vi "TypeConv.vi"(6 "Manifestation Ancestor Path":path, 7 "Action":T2, 8 "Type Path":path, 9 "Alternative Name":string, 10 "Category":T1, 11 "Type Name":string) -> (0 "Has Projection?":bool, 1 "Projection Out":string, 2 "Param Writer":refnum<class "Abstract Param Writer.lvclass">, 3 "Type Path":path, 4 "Queried Category":T1)   [LabVIEW 2013]
uses:
  Action.ctl
  Category.ctl
  Abstract Param Writer/Abstract Param Writer.lvclass
  Bool Writer/Bool Writer.lvclass
  Number Writer/Number Writer.lvclass
  Number Writer/Number Writer.lvclass/Number Writer.ctl
  Number Writer/Numeric Type.ctl
  Enum Writer/Enum Writer.lvclass
  Enum Writer/Enum Writer.lvclass/Enum Writer.ctl
  Simple Struct Writer/Simple Struct Writer.lvclass
  Simple Struct Writer/Simple Struct Writer.lvclass/Simple Struct Writer.ctl
  Opaque Struct Writer/Opaque Struct Writer.lvclass
  Manifestation Writer/Manifestation Writer.lvclass/Manifestation Writer.ctl
  Identity Writer/Identity Writer.lvclass
  String Writer/String Writer.lvclass
  Array Writer/Array Writer.lvclass
  Array Writer/Array Writer.lvclass/Array Writer.ctl
  Manifestation Writer/Manifestation Writer.lvclass
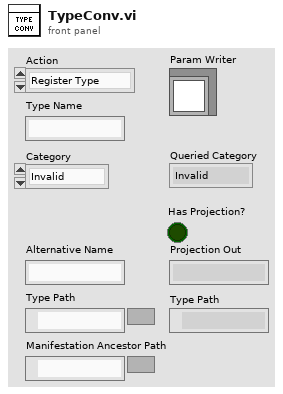
[diagram p1: front panel]
types:
  T1 = typedef "Category.ctl" = enum16{"Invalid", "Void", "Boolean", "Numeric", "Enum", "SimpleStruct", "OpaqueStruct", "SimpleIdentity", "QObject", "SimpleContainer", "FullArray"}
  T2 = typedef "Action.ctl" = enum16{"Register Type", "Register Projection", "Obtain Writer", "Get Projection", "Get Type Path", "Get Type Category"}
  T3 = typedef "Number Writer.lvclass/Numeric Type.ctl" = enum16{"I8", "I16", "I32", "I64", "U8", "U16", "U32", "U64", "SGL", "DBL", "PTR INT", "PTR UINT"}
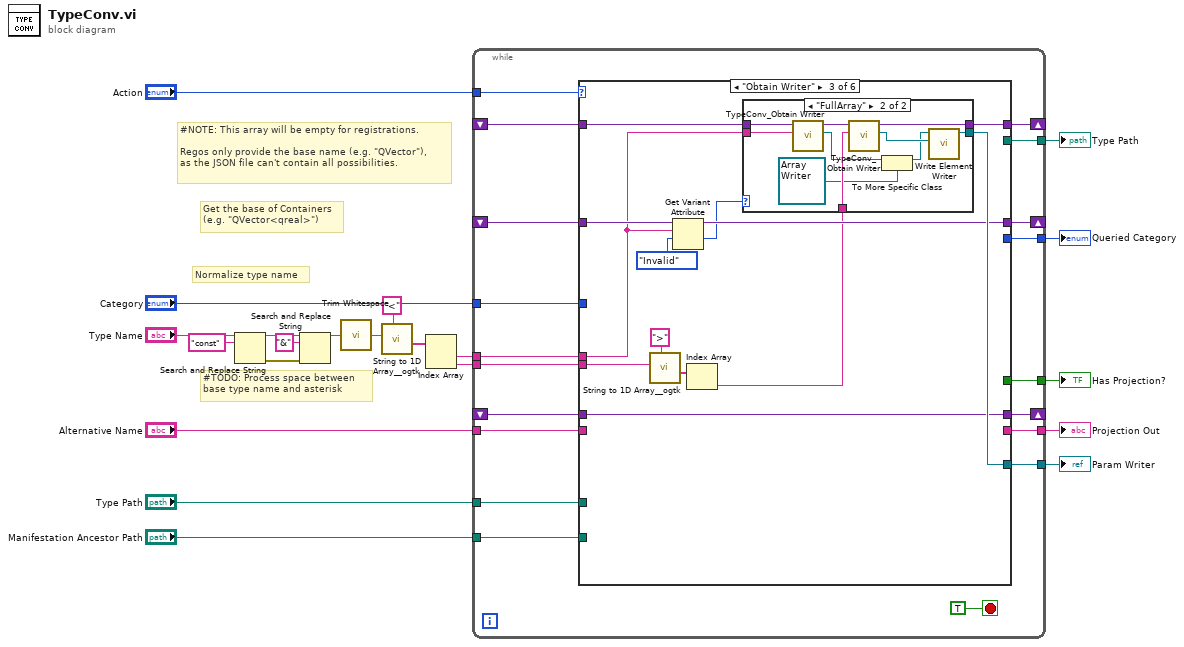
[diagram p0: block diagram]
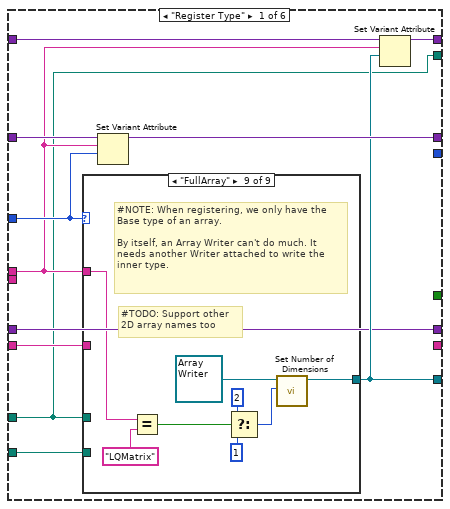
[diagram p2: hidden frame]
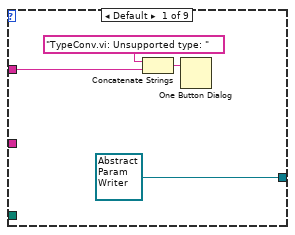
[diagram p3: hidden frame]
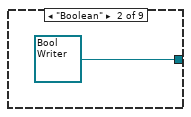
[diagram p4: hidden frame]
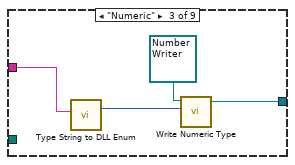
[diagram p5: hidden frame]
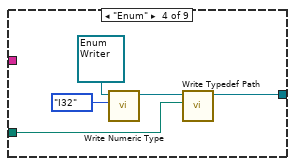
[diagram p6: hidden frame]
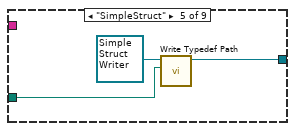
[diagram p7: hidden frame]
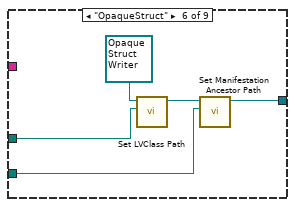
[diagram p8: hidden frame]
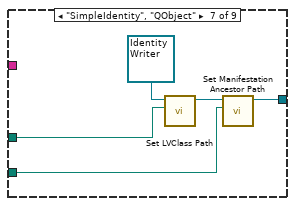
[diagram p9: hidden frame]
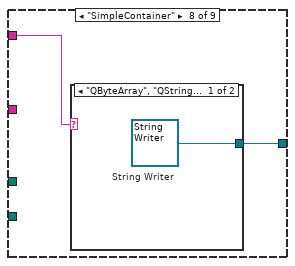
[diagram p10: hidden frame]
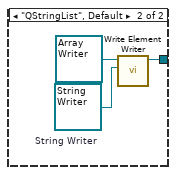
[diagram p11: hidden frame]
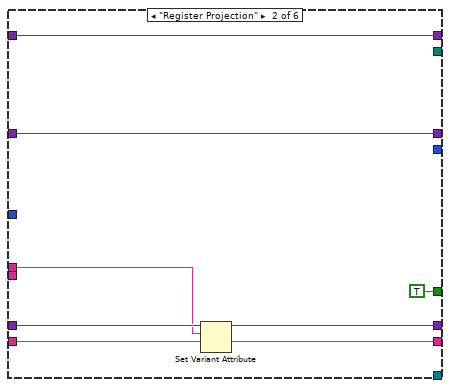
[diagram p12: hidden frame]
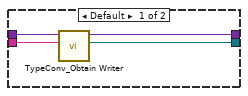
[diagram p13: hidden frame]
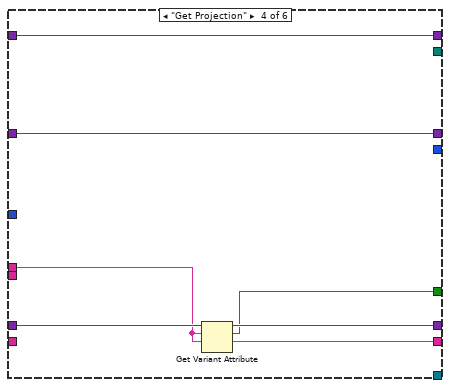
[diagram p14: hidden frame]
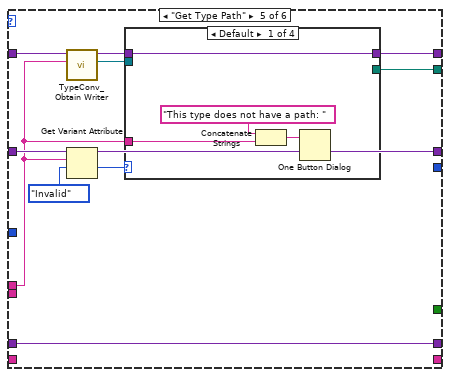
[diagram p15: hidden frame]
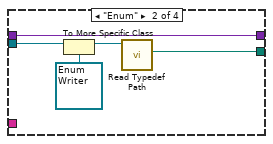
[diagram p16: hidden frame]
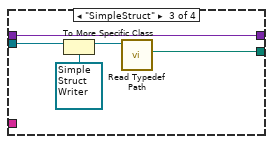
[diagram p17: hidden frame]
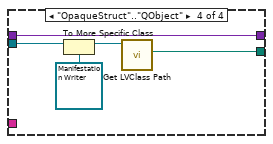
[diagram p18: hidden frame]
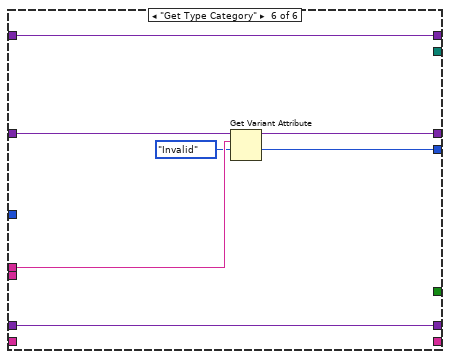
[diagram p19: hidden frame]
diagram:
  # "#NOTE: This array will be empty for registrations.\n\nRegos only provide the base name (e.g. \"QVector\"),\nas the JSON file can't contain all possibilities."
  # "Get the base of Containers\n(e.g. \"QVector<qreal>\")"
  # "#TODO: Process space between\nbase type name and asterisk"
  # "Normalize type name"
  n1 = Search and Replace String(input string="Type Name", search string="const") -> (result string=w18:string, error out=w16:errorcluster)  [unwired: 6 in, 2 out]
  n2 = Search and Replace String(input string=w18, search string="&", error in=w16) -> (result string=w15:string)  [unwired: 5 in, 3 out]
  n3 = call <vilib>:"Trim Whitespace.vi"("string"=w15) -> ("trimmed string"=w9:string)  [unwired: 1 in]
  n4 = call <userlib>:"String to 1D Array__ogtk.vi"("delimiter (Tab)"="<", "string"=w9) -> ("Array of Strings"=w10:string[])  [unwired: 9 in]
  n5 = Index Array(array=w10) -> (element #1=w8:string, element #2=w7:string)  [unwired: 2 in]
  n6 = while {
    tunnel: "Action" -> [w39]
    tunnel: w8 -> [w38]
    shift-right: [w36] -> _
    shift-left: _ -> [w37]
    tunnel: [w35] -> w13
    shift-right: [w33] -> _
    shift-left: _ -> [w34]
    tunnel: "Category" -> [w32]
    tunnel: "Type Path" -> [w31]
    tunnel: w7 -> [w30]
    shift-right: [w28] -> _
    shift-left: _ -> [w27]
    tunnel: "Alternative Name" -> [w29]
    tunnel: [w26] -> w5
    tunnel: [w25] -> w4
    tunnel: "Manifestation Ancestor Path" -> [w24]
    tunnel: [w23] -> w2
    tunnel: [w22] -> w1
    stop <- TRUE stop-if-true
    n7 = case shown="\"Obtain Writer\"" w39 {
      tunnel: w38 -> [w47 w95 w107 w128 w134 w166]
      tunnel: w37 -> [w51 w98 w109 w133 w143 w168]
      tunnel: [w50 w98 w108 w133 w142 w167] -> w36
      tunnel: [w46 _ w110 _ _ _] -> w35
      tunnel: w34 -> [w45 w99 w112 w132 w138 w170]
      tunnel: [w49 w99 w111 w132 w140 w170] -> w33
      tunnel: w32 -> [w48 _ _ _ _ _]
      tunnel: w31 -> [w41 _ _ _ _ _]
      tunnel: w30 -> [_ _ w102 _ _ _]
      tunnel: w29 -> [w42 w94 _ _ _ _]
      tunnel: [w44 w96 w100 w130 w144 w169] -> w28
      tunnel: w27 -> [w44 w97 w100 w131 w144 w169]
      tunnel: [_ w94 _ w129 _ _] -> w26
      tunnel: [_ TRUE _ w127 _ _] -> w25
      tunnel: w24 -> [w43 _ _ _ _ _]
      tunnel: [w41 _ _ _ w135 _] -> w23
      tunnel: [_ _ _ _ _ w164] -> w22
      frame "Register Type" {
        n8 = case shown="\"FullArray\"" w48 {
          tunnel: [refnum<class "Abstract Param Writer.lvclass"> refnum ("Abstract Param Writer.lvclass") refnum<class "Bool Writer.lvclass"> refnum ("Bool Writer.lvclass") w58 w62 w67 w70 w75 w79 w91] -> w46
          tunnel: w47 -> [w53 _ _ _ _ _ _ w80 w90]
          tunnel: w41 -> [_ _ _ w61 w66 w72 w78 _ _]
          tunnel: w43 -> [_ _ _ _ _ w69 w74 _ _]
          tunnel: w42 -> [_ _ w57 _ _ _ _ _ _]
          frame Default {
            n9 = Concatenate Strings("TypeConv.vi: Unsupported type: ", w53) -> (w52:string)
            n10 = One Button Dialog(message=w52) -> ()  [unwired: 1 in, 1 out]
          }
          frame "Boolean" {
          }
          frame "Numeric" {
            n11 = call "Type String to DLL Enum.vi"("Base Numeric Name"=w57) -> ("Numeric Type"=w59:T3)  [unwired: 10 in]
            n12 = call "Write Numeric Type.vi"("Numeric Type"=w59, "Number Writer in"=refnum<class "Number Writer.lvclass"> refnum ("Number Writer.lvclass")) -> ("Number Writer out"=w58:refnum<class "Number Writer.lvclass">)  [unwired: 8 in, 1 out]
          }
          frame "Enum" {
            n13 = call "Write Numeric Type.vi"("Numeric Type"=Numeric_Type."I32", "Number Writer in"=refnum<class "Enum Writer.lvclass"> refnum ("Enum Writer.lvclass")) -> ("Number Writer out"=w63:refnum<class "Enum Writer.lvclass">)  [unwired: 8 in, 1 out]
            n14 = call "Write Typedef Path.vi"("Typedef Path"=w61, "Enum Writer in"=w63) -> ("Enum Writer out"=w62:refnum<class "Enum Writer.lvclass">)  [unwired: 8 in, 1 out]
          }
          frame "SimpleStruct" {
            n15 = call "Write Typedef Path.vi"("Typedef Path"=w66, "Simple Struct Writer in"=refnum<class "Simple Struct Writer.lvclass"> refnum ("Simple Struct Writer.lvclass")) -> ("Simple Struct Writer out"=w67:refnum<class "Simple Struct Writer.lvclass">)  [unwired: 8 in, 1 out]
          }
          frame "OpaqueStruct" {
            n16 = call "Set LVClass Path.vi"("LVClass Path"=w72, "Manifestation Writer in"=refnum<class "Opaque Struct Writer.lvclass"> refnum ("Opaque Struct Writer.lvclass")) -> ("Manifestation Writer out"=w71:refnum<class "Opaque Struct Writer.lvclass">)  [unwired: 9 in]
            n17 = call "Set Manifestation Ancestor Path.vi"("Manifestation Ancestor Path"=w69, "Manifestation Writer in"=w71) -> ("Manifestation Writer out"=w70:refnum<class "Opaque Struct Writer.lvclass">)  [unwired: 9 in]
          }
          frame "SimpleIdentity", "QObject" {
            n18 = call "Set LVClass Path.vi"("LVClass Path"=w78, "Manifestation Writer in"=refnum<class "Identity Writer.lvclass"> refnum ("Identity Writer.lvclass")) -> ("Manifestation Writer out"=w76:refnum<class "Identity Writer.lvclass">)  [unwired: 9 in]
            n19 = call "Set Manifestation Ancestor Path.vi"("Manifestation Ancestor Path"=w74, "Manifestation Writer in"=w76) -> ("Manifestation Writer out"=w75:refnum<class "Identity Writer.lvclass">)  [unwired: 9 in]
          }
          frame "SimpleContainer" {
            n20 = case shown="\"QByteArray\", \"QString\"" w80 {
              tunnel: [w81 w83] -> w79
              frame "QByteArray", "QString" {
                w81 = refnum<class "String Writer.lvclass"> refnum  # String Writer
              }
              frame "QStringList", Default {
                w82 = refnum<class "String Writer.lvclass"> refnum  # String Writer
                n21 = call "Write Element Writer.vi"("Abstract Param Writer.lvclass"=w82, "Array Writer in"=refnum<class "Array Writer.lvclass"> refnum ("Array Writer.lvclass")) -> ("Array Writer out"=w83:refnum<class "Array Writer.lvclass">)  [unwired: 9 in]
              }
            }
          }
          frame "FullArray" {
            # "#TODO: Support other\n2D array names too"
            # "#NOTE: When registering, we only have the\nBase type of an array.\n\nBy itself, an Array Writer can't do much. It \nneeds another Writer attached to write the\ninner type."
            n22 = Equal?(x=w90, y="LQMatrix") -> (x = y?=w88:bool)
            n23 = Select(t=u32 2 ("No. of Dimensions (1)"), s=w88, f=u32 1 ("No. of Dimensions (1)")) -> (s? t:f=w85:u32)
            n24 = call "Set Number of Dimensions.vi"("No. of Dimensions (1)"=w85, "Array Writer in"=refnum<class "Array Writer.lvclass"> refnum ("Array Writer.lvclass")) -> ("Array Writer out"=w91:refnum<class "Array Writer.lvclass">)  [unwired: 9 in]
          }
        }
        n25 = Set Variant Attribute(Variant=w51, name=w47, value=w48) -> (Variant out=w50:variant)  [unwired: 1 in, 2 out]
        n26 = Set Variant Attribute(Variant=w45, name=w47, value=w46) -> (Variant out=w49:variant)  [unwired: 1 in, 2 out]
      }
      frame "Register Projection" {
        n27 = Set Variant Attribute(Variant=w97, name=w95, value=w94) -> (Variant out=w96:variant)  [unwired: 1 in, 2 out]
      }
      frame "Obtain Writer" {
        n28 = call <userlib>:"String to 1D Array__ogtk.vi"("delimiter (Tab)"=">", "string"=w102) -> ("Array of Strings"=w103:string[])  [unwired: 9 in]
        n29 = Get Variant Attribute(Variant=w109, name=w107, default value (empty Variant)=Category."Invalid" ("Category")) -> (duplicate Variant=w108:variant, value=w105:T1)  [unwired: 1 in, 2 out]
        n30 = Index Array(array=w103) -> (element=w101:string)  [unwired: 1 in]
        n31 = case shown="\"FullArray\"" w105 {
          tunnel: w112 -> [w116 w122]
          tunnel: [w115 w126] -> w111
          tunnel: [w114 w124] -> w110
          tunnel: w107 -> [w113 w119]
          tunnel: w101 -> [_ w125]
          frame Default {
            n32 = call "TypeConv_Obtain Writer.vi"("Class Name"=w113, "Writer Map"=w116) -> ("Abstract Param Writer out"=w114:refnum<class "Abstract Param Writer.lvclass">, "Writer Map Dup"=w115:variant)  [unwired: 8 in]
          }
          frame "FullArray" {
            n33 = call "TypeConv_Obtain Writer.vi"("Class Name"=w119, "Writer Map"=w122) -> ("Abstract Param Writer out"=w120:refnum<class "Abstract Param Writer.lvclass">, "Writer Map Dup"=w121:variant)  [unwired: 8 in]
            n34 = call "TypeConv_Obtain Writer.vi"("Class Name"=w125, "Writer Map"=w121) -> ("Abstract Param Writer out"=w123:refnum<class "Abstract Param Writer.lvclass">, "Writer Map Dup"=w126:variant)  [unwired: 8 in]
            n35 = To More Specific Class(target class=refnum<class "Array Writer.lvclass"> refnum ("Array Writer.lvclass"), reference=w120) -> (specific class reference=w117:refnum<class "Array Writer.lvclass">)  [unwired: 1 in, 1 out]
            n36 = call "Write Element Writer.vi"("Abstract Param Writer.lvclass"=w123, "Array Writer in"=w117) -> ("Array Writer out"=w124:refnum<class "Array Writer.lvclass">)  [unwired: 9 in]
          }
        }
      }
      frame "Get Projection" {
        n37 = Get Variant Attribute(Variant=w131, name=w128, default value (empty Variant)=w128) -> (duplicate Variant=w130:variant, found=w127:bool, value=w129:string)  [unwired: 1 in, 1 out]
      }
      frame "Get Type Path" {
        n38 = call "TypeConv_Obtain Writer.vi"("Class Name"=w134, "Writer Map"=w138) -> ("Abstract Param Writer out"=w136:refnum<class "Abstract Param Writer.lvclass">, "Writer Map Dup"=w137:variant)  [unwired: 8 in]
        n39 = Get Variant Attribute(Variant=w143, name=w134, default value (empty Variant)=Category."Invalid" ("Category")) -> (duplicate Variant=w142:variant, value=w139:T1)  [unwired: 1 in, 2 out]
        n40 = case shown="Default" w139 {
          tunnel: w137 -> [w148 w153 w158 w163]
          tunnel: [w148 w153 w158 w163] -> w140
          tunnel: w136 -> [_ w152 w157 w162]
          tunnel: [_ w149 w154 w159] -> w135
          tunnel: w134 -> [w146 _ _ _]
          frame Default {
            n41 = Concatenate Strings("This type does not have a path: " ("string"), w146) -> (w145:string)
            n42 = One Button Dialog(message=w145) -> ()  [unwired: 1 in, 1 out]
          }
          frame "Enum" {
            n43 = To More Specific Class(target class=refnum<class "Enum Writer.lvclass"> refnum ("Enum Writer in"), reference=w152) -> (specific class reference=w150:refnum<class "Enum Writer.lvclass">)  [unwired: 1 in, 1 out]
            n44 = call "Read Typedef Path.vi"("Enum Writer in"=w150) -> ("Typedef Path"=w149:path)  [unwired: 9 in, 1 out]
          }
          frame "SimpleStruct" {
            n45 = To More Specific Class(target class=refnum<class "Simple Struct Writer.lvclass"> refnum ("Enum Writer in"), reference=w157) -> (specific class reference=w155:refnum<class "Simple Struct Writer.lvclass">)  [unwired: 1 in, 1 out]
            n46 = call "Read Typedef Path.vi"("Simple Struct Writer in"=w155) -> ("Typedef Path"=w154:path)  [unwired: 8 in, 2 out]
          }
          frame "OpaqueStruct".."QObject" {
            n47 = To More Specific Class(target class=refnum<class "Manifestation Writer.lvclass"> refnum ("Enum Writer in"), reference=w162) -> (specific class reference=w160:refnum<class "Manifestation Writer.lvclass">)  [unwired: 1 in, 1 out]
            n48 = call "Get LVClass Path.vi"("Manifestation Writer in"=w160) -> ("LVClass Path"=w159:path)  [unwired: 9 in, 1 out]
          }
        }
      }
      frame "Get Type Category" {
        n49 = Get Variant Attribute(Variant=w168, name=w166, default value (empty Variant)=Category."Invalid" ("Category")) -> (duplicate Variant=w167:variant, value=w164:T1)  [unwired: 1 in, 2 out]
      }
    }
  }
  "Param Writer" <- w13
  "Projection Out" <- w5
  "Has Projection?" <- w4
  "Type Path" <- w2
  "Queried Category" <- w1
